vi "down.vi"(3 "Array 2":cluster{"Numeric":dbl, "Numeric 2":dbl}[](array[cluster]), 5 "initialized array":bool[][](array[boolean])) -> (0 "x = y?":bool, 1 "appended array":cluster{"Numeric":dbl, "Numeric 2":dbl}[](array[cluster]), 2 "Array 3":bool[][](array[boolean]))   [LabVIEW 2009]
uses:
  Global 3.vi
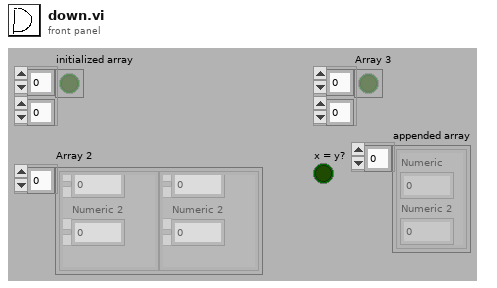
[diagram p1: front panel]
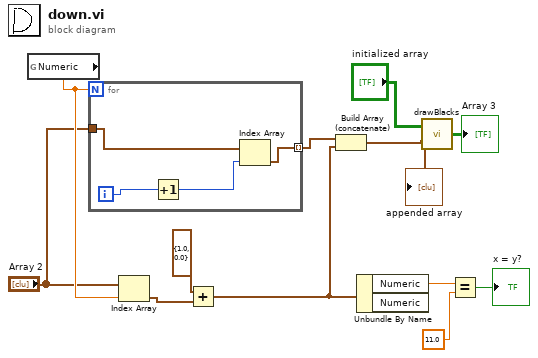
[diagram p0: block diagram]
diagram:
  n1 = global read "Global 3.vi" "Numeric"() -> (w2:dbl)
  n2 = for {
    N: w2 -> [_]
    tunnel: "Array 2" -> [w16]
    tunnel: [w13] -> w5 mode=indexing
    i -> [w15]
    n3 = Increment(x=w15) -> (x+1=w14:i32)
    n4 = Index Array(array=w16, index=w14) -> (element=w13:cluster{"Numeric":dbl, "Numeric 2":dbl})
  }
  n5 = Index Array(array="Array 2", index=w2) -> (element=w3:cluster{"Numeric":dbl, "Numeric 2":dbl})
  n6 = Add(x=cluster{"Numeric":dbl, "Numeric 2":dbl} {"Numeric"=1.0, "Numeric 2"=0.0}, y=w3) -> (x+y=w9:cluster{"Numeric":dbl, "Numeric 2":dbl})
  n7 = Build Array (concatenate)(w5, w9) -> (w6:cluster{"Numeric":dbl, "Numeric 2":dbl}[])
  "appended array" <- w6
  n8 = Unbundle By Name(w9) -> ("Numeric"=w10:dbl)  [unwired: 1 out]
  n9 = call "drawBlacks.vi"("Array 2"=w6, "Array 3"="initialized array") -> ("Array"=→"Array 3":bool[][])
  n10 = Equal?(x=w10, y=11.0) -> (x = y?=→"x = y?":bool)
